vi "Create Async Threads.vi"(8 "error in (no error)":errorcluster, 10 "Transfer Groups":refnum<class "Transfer Group.lvclass">[](array[class]), 11 "Plugin in":refnum<class "Plugin.lvclass">) -> (0 "error out":errorcluster, 3 "Plugin out":refnum<class "Plugin.lvclass">)   [LabVIEW 2017, in "DSF Core.lvlib" / "Plugin.lvclass"]
uses:
  Plugin.lvclass
  Transfer Group/Transfer Group.lvclass
  Buffer Converter/Buffer Converter.lvclass
  Transceiver/Transceiver.lvclass
  Transceiver/Plugin Thread.lvclass
  Plugin.lvclass/Plugin.ctl
panel:
  out "Plugin Thread out":refnum<class "Plugin Thread.lvclass">
  in  "Transceiver":refnum<class "Transceiver.lvclass">
  in  "Buffer Converter":refnum<class "Buffer Converter.lvclass">
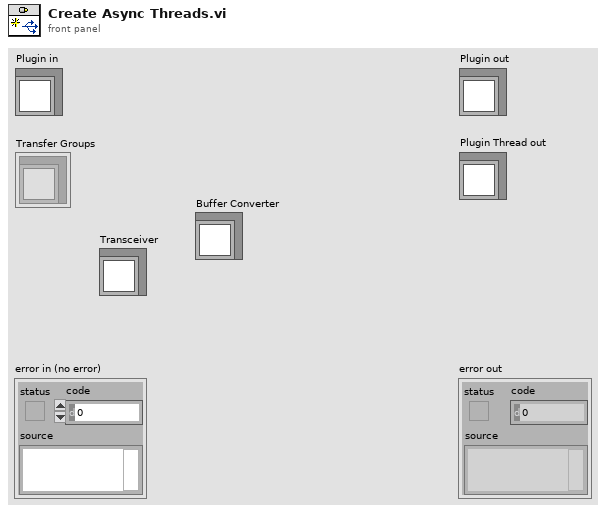
[diagram p1: front panel]
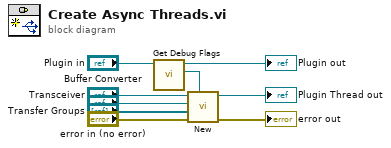
[diagram p0: block diagram]
diagram:
  n1 = call "Get Debug Flags.vi"("Plugin in"="Plugin in") -> ("Debug Flags"=w5:refnum<class "Debug Flags.lvclass">, "Plugin out"=→"Plugin out":refnum<class "Plugin.lvclass">)  [unwired: 9 in]
  n2 = call "New.vi"("Debug Flags"=w5, "error in (no error)"="error in (no error)", "Transfer Groups"="Transfer Groups", "Buffer Converter"="Buffer Converter", "Transceiver"="Transceiver") -> ("error out"=→"error out":errorcluster, "Plugin Thread out"=→"Plugin Thread out":refnum<class "Plugin Thread.lvclass">)  [unwired: 5 in]
